vi "AddFilterToTree.vi"(4 "Category Priorities":i32[](array[numeric]), 6 "Category Names":string[](array[string]), 10 "Filter":string, 11 "Tree Refnum In":refnum<vi>) -> (3 "Tree Refnum Out":refnum<vi>)   [LabVIEW 2016, in "NI_NPW_Filters.lvlib"]
uses:
  <resource>/dialog/NewProjectWizard/Filters/NI_NPW_Filters.lvlib
panel:
  in  "Test Tree":string(tree)
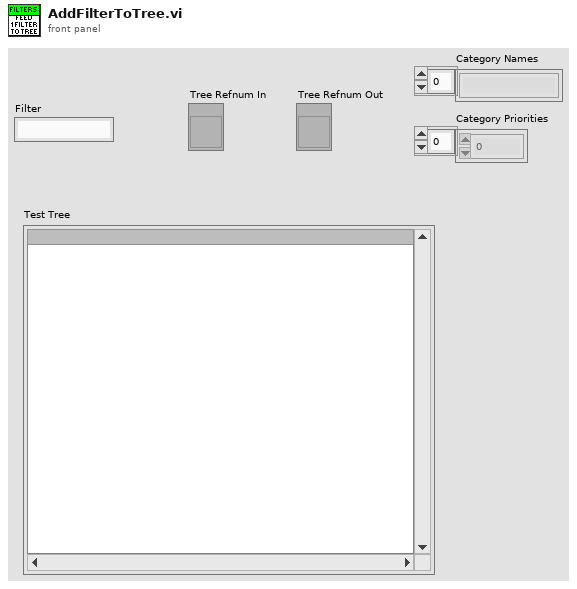
[diagram p1: front panel]
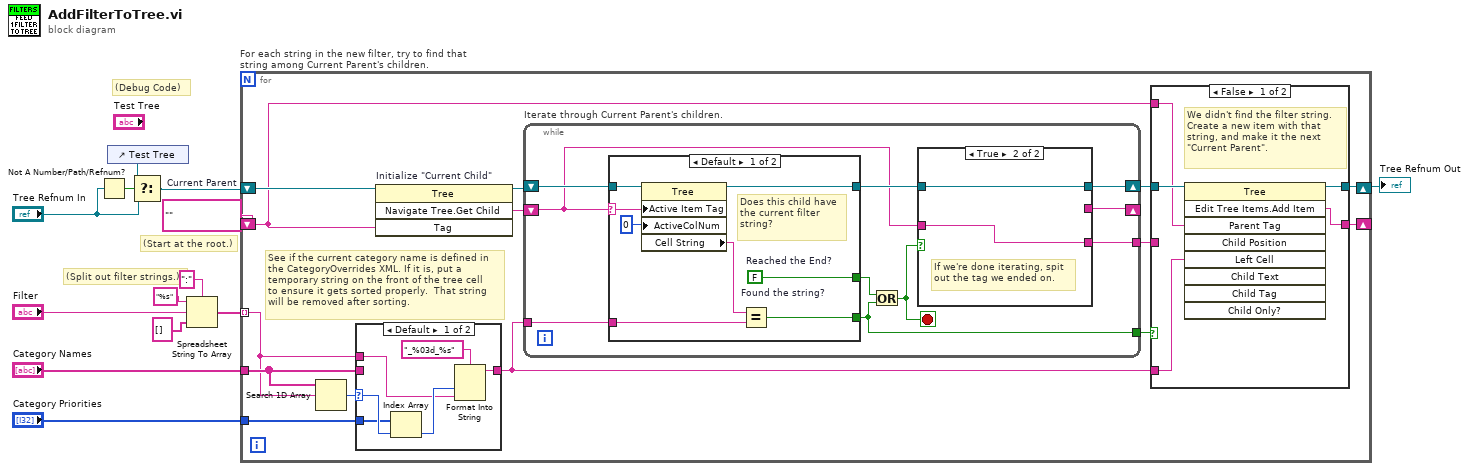
[diagram p0: block diagram]
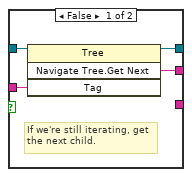
[diagram p4: hidden frame]
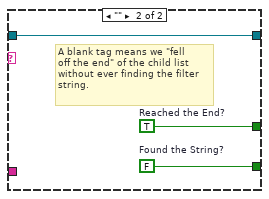
[diagram p5: hidden frame]
diagram:
  w9 = ""  # Current Parent
  # "(Split out filter strings.)"
  # "(Start at the root.)"
  # "(Debug Code)"
  n1 = Not A Number/Path/Refnum?(number/path/refnum="Tree Refnum In") -> (NaN/Path/Refnum?=w4:bool)
  n2 = control-ref of="Test Tree"() -> (w7:refnum<vi>)
  n3 = Select(t=w7, s=w4, f="Tree Refnum In") -> (s? t:f=w6:refnum<vi>)
  n4 = Spreadsheet String To Array(delimiter (Tab)=":", format string="%s", spreadsheet string="Filter", array type (2D Dbl)=string[] []) -> (array=w10:string[])
  n5 = for "For each string in the new filter, try to find that string among Current Parent's children." {
    tunnel: w10 -> [w14] mode=indexing
    shift-right: [w26] -> _
    shift-left: w9 -> [w22]
    shift-right: [w25] -> w5
    shift-left: w6 -> [w24]
    tunnel: "Category Names" -> [w17]
    tunnel: "Category Priorities" -> [w16]
    # "See if the current category name is defined in the CategoryOverrides XML. If it is, put a temporary string on the front of the tree cell\nto ensure it gets sorted properly.  That string will be removed after sorting."
    n6 = Search 1D Array(1D array=w17, element=w14) -> (index of element=w18:i32)  [unwired: 1 in]
    n7 = case shown="Default" w18 {
      selector: w18 -> [w33 _]
      tunnel: w17 -> [_ _]
      tunnel: [w29 w34] -> w15
      tunnel: w16 -> [w32 _]
      tunnel: w14 -> [w28 w34]
      frame Default {
        n8 = Index Array(array=w32, index=w33) -> (element=w30:i32)
        n9 = Format Into String(format string="_%03d_%s", w30, w28) -> (resulting string=w29:string)  [unwired: 2 in, 1 out]
      }
      frame -1 {
      }
    }
    n10 = invoke on="Initialize \"Current Child\"" class="Tree" method="Navigate Tree.Get Child"(reference=w24, "Tag"=w22) -> (reference out=w23:refnum<vi>, "Navigate Tree:Get Child"=w21:string)  [unwired: 2 in, 2 out]
    n11 = while "Iterate through Current Parent's children." {
      shift-right: [w46] -> _
      shift-left: w21 -> [w44]
      tunnel: w15 -> [w51]
      shift-right: [w47] -> w27
      shift-left: w23 -> [w50]
      tunnel: [w43] -> w20
      tunnel: [w42] -> w19
      stop <- w49 stop-if-true
      n12 = case shown="Default" w44 {
        selector: w44 -> [w58 _]
        tunnel: w50 -> [w65 w68]
        tunnel: w51 -> [w62 _]
        tunnel: [w61 w67] -> w43
        tunnel: [w60 w68] -> w48
        tunnel: [w59 w66] -> w45
        frame Default {
          w59 = FALSE  # Reached the End?
          # "Does this child have\nthe current filter\nstring?"
          n13 = property class="Tree"(reference=w65, "Active Item Tag"=w58, "ActiveColNum"=0 ("Active Cell:Active Column Number")) -> (reference out=w60:refnum<vi>, "Cell String"=w63:string)  [unwired: 1 in, 1 out]
          n14 = Equal? "Found the string?"(x=w63, y=w62) -> (x = y?=w61:bool)
        }
        frame "" {
          w66 = TRUE  # Reached the End?
          w67 = FALSE  # Found the String?
          # "A blank tag means we \"fell\noff the end\" of the child list\nwithout ever finding the filter\nstring."
        }
      }
      n15 = Or(x=w45, y=w43) -> (x .or. y?=w49:bool)
      n16 = case "If we're still iterating, get the next child." shown="True" w49 {
        tunnel: w48 -> [w55 w57]
        tunnel: [w54 w57] -> w47
        tunnel: w44 -> [w53 w56]
        tunnel: [w52 _] -> w46
        tunnel: [_ w56] -> w42
        frame False {
          # "If we're still iterating, get\nthe next child."
          n17 = invoke class="Tree" method="Navigate Tree.Get Next"(reference=w55, "Tag"=w53) -> (reference out=w54:refnum<vi>, "Navigate Tree:Get Next Item"=w52:string)  [unwired: 2 in, 2 out]
        }
        frame True {
          # "If we're done iterating, spit\nout the tag we ended on."
        }
      }
    }
    n18 = case shown="False" w20 {
      tunnel: w22 -> [w37 _]
      tunnel: w27 -> [w39 w41]
      tunnel: [w38 w40] -> w26
      tunnel: w15 -> [w35 _]
      tunnel: [w36 w41] -> w25
      tunnel: w19 -> [_ w40]
      frame False {
        # "We didn't find the filter string.\nCreate a new item with that\nstring, and make it the next\n\"Current Parent\"."
        n19 = invoke class="Tree" method="Edit Tree Items.Add Item"(reference=w39, "Parent Tag"=w37, "Left Cell"=w35) -> (reference out=w36:refnum<vi>, "Edit Tree Items:Add Item"=w38:string)  [unwired: 6 in, 7 out]
      }
      frame True {
        # "We found an item with the\ncurrent filter string!\n\nIt becomes the \"Current Parent\"\nfor the next iteration."
      }
    }
  }
  "Tree Refnum Out" <- w5
